vi "Add Crosshairs to image.vi"(6 "Color":u32(colorbox)=15664896, 7 "Show Crosshairs":bool=TRUE, 8 "error in":errorcluster, 11 "Image In":T1) -> (0 "error out":errorcluster, 3 "Image Out":T1)   [LabVIEW 2013]
doc: "This Optionally adds a salbar as an overlay to an Image Buffer.\nThe pixel size in um is required.s"
uses:
  <vilib>/vision/Image Controls.llb/IMAQ Image.ctl
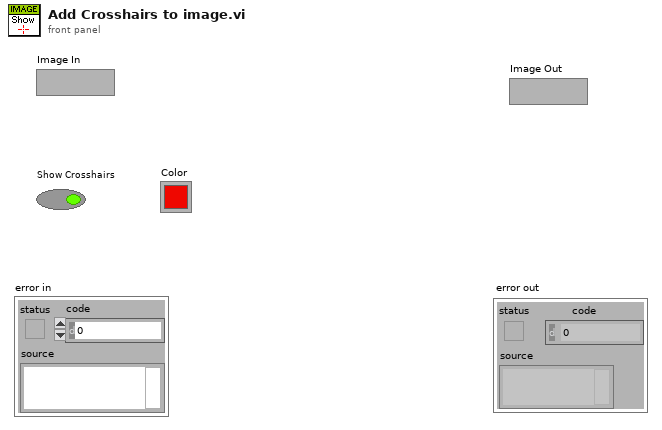
[diagram p1: front panel]
types:
  T1 = typedef "IMAQ Image.ctl" = refnum<image>
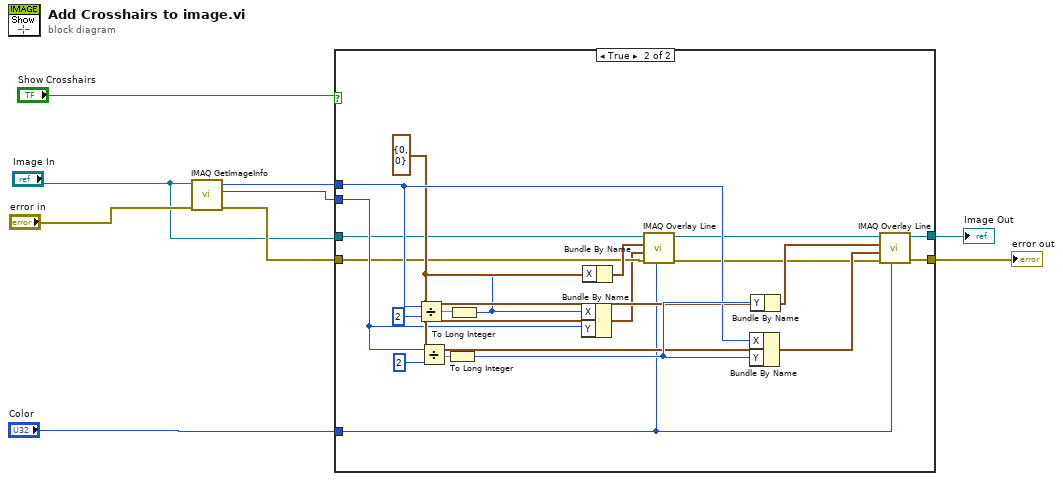
[diagram p0: block diagram]
diagram:
  n1 = call "IMAQ GetImageInfo"("error in (no error)"="error in", "Image"="Image In") -> ("error out"=w5:errorcluster, "Y Resolution"=w6:i32, "X Resolution"=w7:i32)  [unwired: 2 in, 5 out]
  n2 = case shown="True" "Show Crosshairs" {
    tunnel: [w10 w28] -> w9
    tunnel: "Image In" -> [w11 w17]
    tunnel: w5 -> [w10 w16]
    tunnel: [w11 w29] -> w3
    tunnel: w7 -> [_ w24]
    tunnel: w6 -> [_ w19]
    tunnel: "Color" -> [_ w15]
    frame False {
    }
    frame True {
      w21 = cluster{"X":i32, "Y":i32} {"X"=0, "Y"=0} ("Start Point")
      n3 = Divide(x=w24, y=2) -> (x/y=w25:dbl)
      n4 = Divide(x=w19, y=2) -> (x/y=w27:dbl)
      n5 = To Long Integer(number=w27) -> (32bit integer=w26:i32)
      n6 = To Long Integer(number=w25) -> (32bit integer=w20:i32)
      n7 = Bundle By Name(cluster=w21, "X"=w20, "Y"=w19) -> (w12:cluster{"X":i32, "Y":i32})
      n8 = Bundle By Name(cluster=w21, "X"=w20) -> (w18:cluster{"X":i32, "Y":i32})
      n9 = call "IMAQ Overlay Line"("Color"=w15, "error in (no error)"=w16, "End Point"=w12, "Start Point"=w18, "Image"=w17) -> ("error out"=w13:errorcluster, "Image Out"=w14:T1)  [unwired: 1 in, 4 out]
      n10 = Bundle By Name(cluster=w21, "X"=w24, "Y"=w26) -> (w22:cluster{"X":i32, "Y":i32})
      n11 = Bundle By Name(cluster=w21, "Y"=w26) -> (w23:cluster{"X":i32, "Y":i32})
      n12 = call "IMAQ Overlay Line"("Color"=w15, "error in (no error)"=w13, "End Point"=w22, "Start Point"=w23, "Image"=w14) -> ("error out"=w28:errorcluster, "Image Out"=w29:T1)  [unwired: 1 in, 4 out]
    }
  }
  "error out" <- w9
  "Image Out" <- w3
